vi "nominal ingest job wait.vi"(7 "out_job":i32, 8 "error in (no error)":errorcluster, 9 "poll_interval_ms":dbl, 10 "rid":string, 11 "client":i32) -> (0 "error out":errorcluster, 3 "function return":i32, 5 "out_job out":i32)   [LabVIEW 2020, in "client.lvlib"]
doc: "int32_t nominal_ingest_job_wait(int32_t client,\n const char *rid,\n double poll_interval_ms,\n int32_t *out_job);"
uses:
  client.lvlib
  bin/nominalClient_64.dll
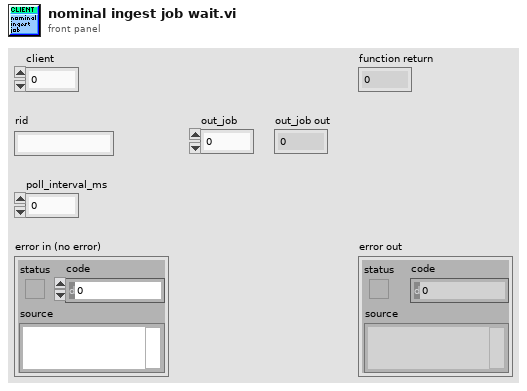
[diagram p1: front panel]
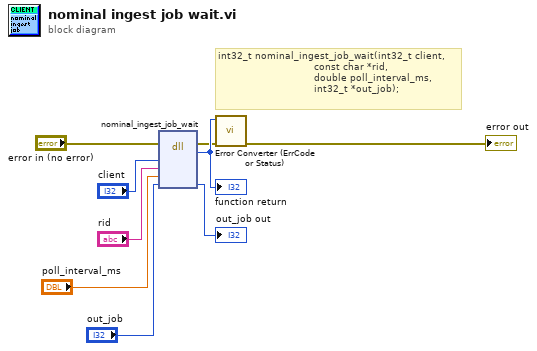
[diagram p0: block diagram]
diagram:
  # "int32_t nominal_ingest_job_wait(int32_t client,\n                                const char *rid,\n                                double poll_interval_ms,\n                                int32_t *out_job);"
  n1 = dll-call lib="C:/code/labview-client-rs/lv_src/bin/nominalClient_*.*" fn="nominal_ingest_job_wait"(error in="error in (no error)", "client"="client", "rid"="rid", "poll_interval_ms"="poll_interval_ms", "out_job"="out_job") -> (error out=w2:errorcluster, w9:i32, "out_job"=→"out_job out":i32)  [unwired: 5 in, 1 out]
  "function return" <- w9
  n2 = call "Error Converter (ErrCode or Status).vi"("error in (no error)"=w2, "error code"=w9) -> ("error out"=→"error out":errorcluster)  [unwired: 9 in]
